vi "GetType.vi"(8 "error in (no error)":errorcluster, 11 "Configure Data Marker [DM] Msg":refnum<class "Configure Data Marker [DM] Msg.lvclass">) -> (0 "error out":errorcluster, 2 "Data Sample":variant, 3 "Configure Data Marker [DM] Msg":refnum<class "Configure Data Marker [DM] Msg.lvclass">)   [LabVIEW 2015, in "CS++Fgen.lvlib" / "Configure Data Marker [DM] Msg.lvclass"]
doc: "This VI delivers a sample of the data type format the message expects."
uses:
  Configure Data Marker [DM] Msg.lvclass
  Configure Data Marker [DM] Msg.lvclass/Configure Data Marker [DM] Msg.ctl
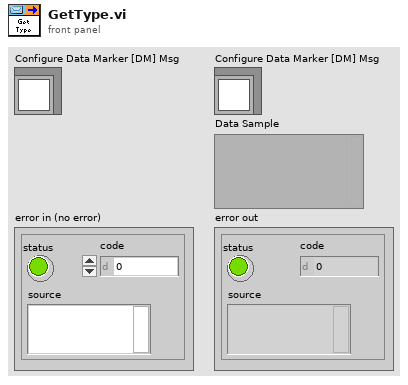
[diagram p1: front panel]
types:
  T1 = cluster{"Source Channel (\"\")":string, "Marker Name (\"\")":string, "Bit Position":i32, "Destination Terminal (None)":string}
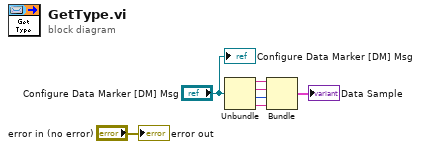
[diagram p0: block diagram]
diagram:
  n1 = Unbundle("Configure Data Marker [DM] Msg") -> (w4:string, w3:string, w2:i32, w1:string)
  n2 = Bundle("Source Channel (\"\")"=w4, "Marker Name (\"\")"=w3, "Bit Position"=w2, "Destination Terminal (None)"=w1) -> (→"Data Sample":T1)  [unwired: 1 in]
  "error out" <- "error in (no error)"
  "Configure Data Marker [DM] Msg" <- "Configure Data Marker [DM] Msg"
